vi "TEST_ASIC_SUMnADDS_(OLD).vi"(7 "Serial Number":string, 8 "error in":errorcluster, 11 "Instrument VISA in":T1={"AWG VISA"="generadorpulsos", "Oscilloscope  VISA "="Oscilloscope", "Integration Board IP"="172.16.7.43", "connection ID"=refnum, "report out"=refnum, "report file path"=path "C:/Documents and Settings/CTA_LAB01/Desktop/L0_Asic/L0 Asic Test Data"}) -> (0 "error out":errorcluster, 3 "Instrument VISA out":T1={"AWG VISA"="generadorpulsos", "Oscilloscope  VISA "="Oscilloscope", "Integration Board IP"="172.16.7.43", "connection ID"=refnum, "report out"=refnum, "report file path"=path "C:/Documents and Settings/CTA_LAB01/Desktop/L0_Asic/L0 Asic Test Data"})   [LabVIEW 2009]
uses:
  <vilib>/Utility/NIReport.llb/NI_report.lvclass
  <vilib>/Utility/NIReport.llb/HTML/NI_HTML.lvclass
panel:
  in  "channel array":i32[](array[numeric])=[0, 1, 2, 3, 4, 5, 6]
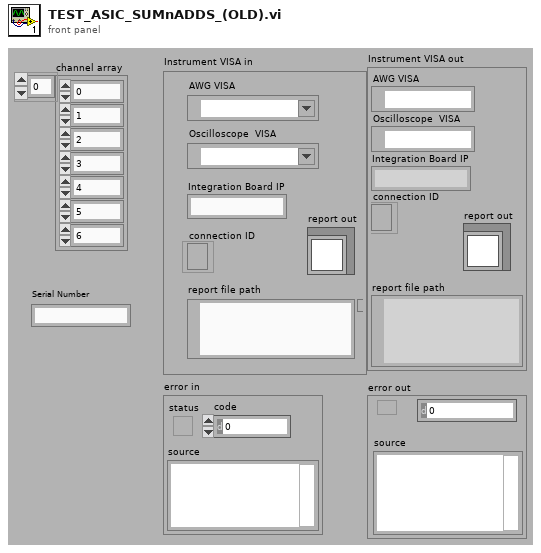
[diagram p1: front panel]
types:
  T1 = cluster{"AWG VISA":refnum<visa-resource-name>, "Oscilloscope  VISA ":refnum<visa-resource-name>, "Integration Board IP":string, "connection ID":refnum<k5>, "report out":refnum<class "NI_report.lvclass">, "report file path":path}
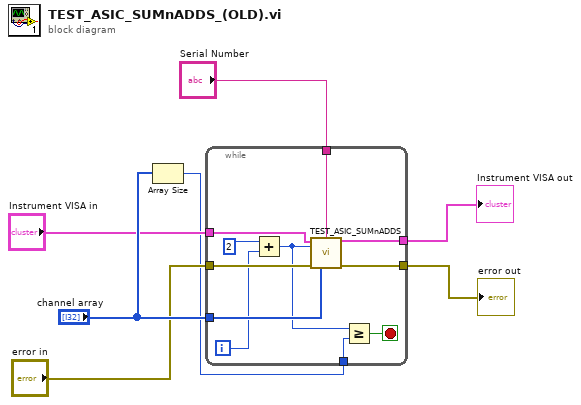
[diagram p0: block diagram]
diagram:
  n1 = Array Size(array="channel array") -> (size(s)=w1:i32)
  n2 = while {
    tunnel: "channel array" -> [w18]
    tunnel: "error in" -> [w17]
    tunnel: [w16] -> w5
    tunnel: [w15] -> w4
    tunnel: "Instrument VISA in" -> [w14]
    tunnel: "Serial Number" -> [w13]
    tunnel: w1 -> [w10]
    i -> [w9]
    stop <- w11 stop-if-true
    n3 = Add(x=2, y=w9) -> (x+y=w8:i32)
    n4 = call "TEST_ASIC_SUMnADDS.vi"("Instrument VISA in"=w14, "Serial number"=w13, "quantity"=w8, "error in"=w17, "channel array"=w18) -> ("Instrument VISA out"=w15:T1, "error out"=w16:errorcluster)  [unwired: 9 in]
    n5 = Greater Or Equal?(x=w8, y=w10) -> (x >= y?=w11:bool)
  }
  "error out" <- w5
  "Instrument VISA out" <- w4
